vi "Teleop.vi"(10 "Match Info":T1={"Autonomous Elapsed Seconds"=0.0, "TeleOp Elapsed Seconds"=0.0, "Disabled Elapsed Seconds"=0.0, "Visited Autonomous"=FALSE, "Visited TeleOp"=FALSE, "Visited Disabled"=FALSE, "Autonomous Settings"={"Autonomous Style"=enum."Independent", "VI Refnum"=refnum}}, 11 "Call Context":T2) -> ()   [LabVIEW 2013]
doc: "This VI is called for each TeleOp packet received from the DS where the robot is not disabled. It is often used to read from the joysticks and update I/O or to update setpoints for timed control loops. It should complete and return within 20 milliseconds or it may miss DS packets."
uses:
  <vilib>/Rock Robotics/WPI/DriverStation/WPI_DriverStationDerivedRobotMode.ctl
  <vilib>/Rock Robotics/WPI/DriverStation/WPI_DriverStationMatch Info.ctl
  Robot Global Data.vi
  <vilib>/Rock Robotics/WPI/Joystick/WPI_JoystickGetSetRefNum.vi
  <vilib>/Rock Robotics/WPI/RobotDrive/WPI_RobotDriveMecanumDrive_Cartesian.vi
panel:
  in  "slow mode turn multiplier":dbl(knob)=0.5 scale=0.0..1.0
  in  "Deadzone":dbl=0.05
  out "Numeric 1":dbl(slide) scale=0.0..100.0
  out "Boolean 2":bool
  out "Boolean 1":bool
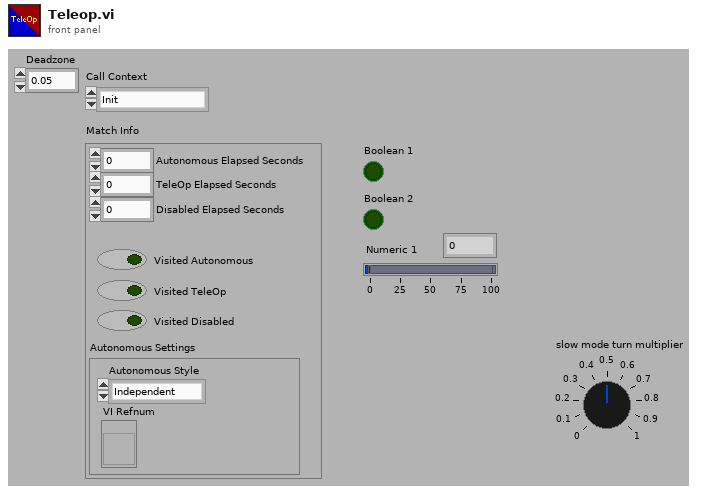
[diagram p1: front panel]
types:
  T1 = typedef "WPI_DriverStationMatch Info.ctl" = cluster{"Autonomous Elapsed Seconds":dbl, "TeleOp Elapsed Seconds":dbl, "Disabled Elapsed Seconds":dbl, "Visited Autonomous":bool, "Visited TeleOp":bool, "Visited Disabled":bool, "Autonomous Settings":cluster{"Autonomous Style":enum16{"Iterative", "Independent"}, "VI Refnum":refnum<vi>}}
  T2 = typedef "WPI_DriverStationDerivedRobotMode.ctl" = enum16{"Init", "Execute", "Stop"}
  T3 = typedef "WPI_JoystickDevRef.ctl" = cluster{"Device":T4}
  T4 = typedef "WPI_JoystickDeviceEnum.ctl" = enum16{"USB 1", "USB 2", "USB 3", "USB 4", "Kinect 1", "Kinect 2"}
  T5 = typedef "WPI_JoystickButtonState.ctl" = cluster{"Button 1":bool, "Button 2":bool, "Button 3":bool, "Button 4":bool, "Button 5":bool, "Button 6":bool, "Button 7":bool, "Button 8":bool, "Button 9":bool, "Button 10":bool, "Button 11":bool, "Button 12":bool}
  T6 = cluster{"axis 1 (x)":dbl, "axis 2 (y)":dbl, "axis 3 (throttle)":dbl, "axis 4":dbl, "axis 5":dbl, "axis 6":dbl}
  T7 = typedef "WPI_RobotDriveDevRef.ctl" = cluster{"DevStatus":errorcluster, "Motors[]":T8[], "Square Inputs":bool, "Max Output":dbl, "Isochronous":bool}
  T8 = typedef "WPI_MotorControlDeviceRef.ctl" = cluster{"DeviceStatus":errorcluster, "Type":enum16{"PWM", "CAN"}, "PWM":cluster{"Digital Module":T9, "PWM Channel":T10, "DeadBand":T11}, "CAN":cluster{"Device Number":u8, "Control Mode":T12, "Semaphore":T13, "Max Vout":dbl}, "Invert":bool, "TransformRef":T14, "InvTransformRef":T14}
  T9 = typedef "FPGA_TypedefDigitalModule.ctl" = enum16{"Digital Module 1", "Digital Module 2"}
  T10 = typedef "FPGA_DIOPWMChannel.ctl" = enum8{"PWM 1", "PWM 2", "PWM 3", "PWM 4", "PWM 5", "PWM 6", "PWM 7", "PWM 8", "PWM 9", "PWM 10", "Invalid"}
  T11 = typedef "WPI_PWMDeadband.ctl" = cluster{"Name":string, "maxPositivePwm":i32, "minPositivePwm":i32, "centerPwm":i32, "maxNegativePwm":i32, "minNegativePwm":i32, "angularRange":u16}
  T12 = typedef "WPI_CANJaguar_ControlMode.ctl" = enum8{"Percent VBus", "Current", "Speed", "Position", "Voltage"}
  T13 = typedef "Semaphore RefNum" = refnum<k1>
  T14 = typedef "WPI_PWMTransform_ConPane.ctl" = refnum<vi>
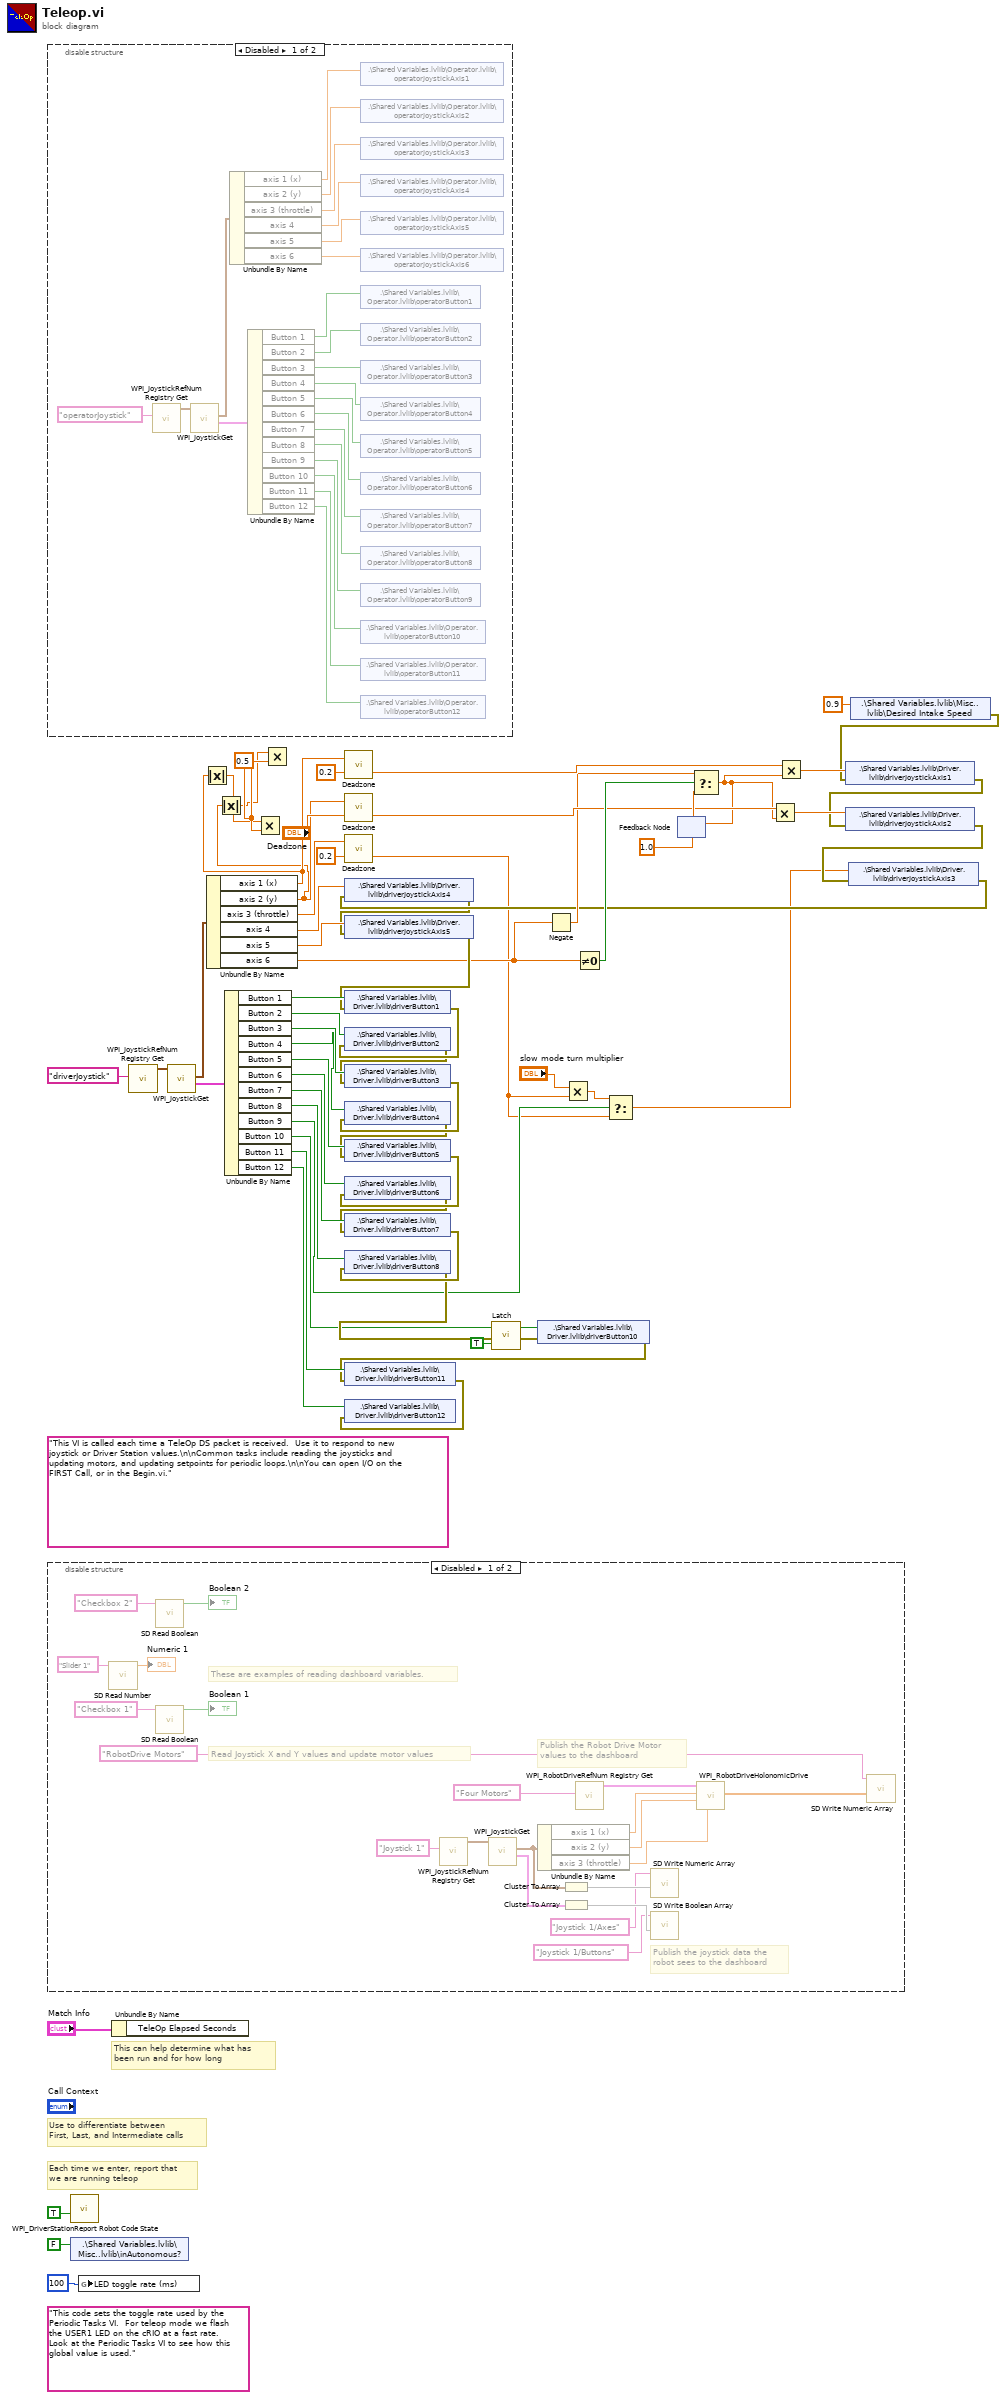
[diagram p0: block diagram]
diagram:
  w4 = 0.5 ("y")
  (unwired) "This code sets the toggle rate used by the Periodic Tasks VI.  For teleop mode we flash the USER1 LED on the cRIO at a fast rate.  Look at the Periodic Tasks VI to see how this global value is used."
  (unwired) "This VI is called each time a TeleOp DS packet is received.  Use it to respond to new joystick or Driver Station values.\n\nCommon tasks include reading the joysticks and updating motors, and updating setpoints for periodic loops.\n\nYou can open I/O on the FIRST Call, or in the Begin.vi."
  # "Each time we enter, report that\nwe are running teleop"
  # "Use to differentiate between\nFirst, Last, and Intermediate calls"
  # "This can help determine what has\nbeen run and for how long"
  n1 = disable-structure shown="Disabled" {
    frame Disabled {
      n2 = call <vilib>:"WPI_JoystickRefNum Registry Get.vi"("refnum name"="operatorJoystick") -> ("JoystickDevRef"=w85:T3)  [unwired: 9 in, 1 out]
      n3 = call <vilib>:"WPI_JoystickGet.vi"("JoystickDevRef"=w85) -> ("Buttons"=w83:T5, "Axes"=w84:T6)  [unwired: 4 in, 1 out]
      n4 = Unbundle By Name(w84) -> ("axis 1 (x)"=w82:dbl, "axis 2 (y)"=w81:dbl, "axis 3 (throttle)"=w80:dbl, "axis 4"=w79:dbl, "axis 5"=w78:dbl, "axis 6"=w77:dbl)
      n5 = Unbundle By Name(w83) -> ("Button 1"=w76:bool, "Button 2"=w75:bool, "Button 3"=w74:bool, "Button 4"=w73:bool, "Button 5"=w72:bool, "Button 6"=w71:bool, "Button 7"=w70:bool, "Button 8"=w69:bool, "Button 9"=w68:bool, "Button 10"=w67:bool, "Button 11"=w66:bool, "Button 12"=w65:bool)
      n6 = shared-variable ".\\Shared Variables.lvlib\\Operator.lvlib\\operatorJoystickAxis1"(w82) -> ()  [unwired: 1 in, 1 out]
      n7 = shared-variable ".\\Shared Variables.lvlib\\Operator.lvlib\\operatorJoystickAxis2"(w81) -> ()  [unwired: 1 in, 1 out]
      n8 = shared-variable ".\\Shared Variables.lvlib\\Operator.lvlib\\operatorJoystickAxis3"(w80) -> ()  [unwired: 1 in, 1 out]
      n9 = shared-variable ".\\Shared Variables.lvlib\\Operator.lvlib\\operatorJoystickAxis4"(w79) -> ()  [unwired: 1 in, 1 out]
      n10 = shared-variable ".\\Shared Variables.lvlib\\Operator.lvlib\\operatorJoystickAxis5"(w78) -> ()  [unwired: 1 in, 1 out]
      n11 = shared-variable ".\\Shared Variables.lvlib\\Operator.lvlib\\operatorJoystickAxis6"(w77) -> ()  [unwired: 1 in, 1 out]
      n12 = shared-variable ".\\Shared Variables.lvlib\\Operator.lvlib\\operatorButton1"(w76) -> ()  [unwired: 1 in, 1 out]
      n13 = shared-variable ".\\Shared Variables.lvlib\\Operator.lvlib\\operatorButton2"(w75) -> ()  [unwired: 1 in, 1 out]
      n14 = shared-variable ".\\Shared Variables.lvlib\\Operator.lvlib\\operatorButton3"(w74) -> ()  [unwired: 1 in, 1 out]
      n15 = shared-variable ".\\Shared Variables.lvlib\\Operator.lvlib\\operatorButton4"(w73) -> ()  [unwired: 1 in, 1 out]
      n16 = shared-variable ".\\Shared Variables.lvlib\\Operator.lvlib\\operatorButton5"(w72) -> ()  [unwired: 1 in, 1 out]
      n17 = shared-variable ".\\Shared Variables.lvlib\\Operator.lvlib\\operatorButton6"(w71) -> ()  [unwired: 1 in, 1 out]
      n18 = shared-variable ".\\Shared Variables.lvlib\\Operator.lvlib\\operatorButton7"(w70) -> ()  [unwired: 1 in, 1 out]
      n19 = shared-variable ".\\Shared Variables.lvlib\\Operator.lvlib\\operatorButton8"(w69) -> ()  [unwired: 1 in, 1 out]
      n20 = shared-variable ".\\Shared Variables.lvlib\\Operator.lvlib\\operatorButton9"(w68) -> ()  [unwired: 1 in, 1 out]
      n21 = shared-variable ".\\Shared Variables.lvlib\\Operator.lvlib\\operatorButton10"(w67) -> ()  [unwired: 1 in, 1 out]
      n22 = shared-variable ".\\Shared Variables.lvlib\\Operator.lvlib\\operatorButton11"(w66) -> ()  [unwired: 1 in, 1 out]
      n23 = shared-variable ".\\Shared Variables.lvlib\\Operator.lvlib\\operatorButton12"(w65) -> ()  [unwired: 1 in, 1 out]
    }
    frame Enabled {
    }
  }
  n24 = disable-structure shown="Disabled" {
    frame Disabled {
      # "These are examples of reading dashboard variables."
      # "Publish the Robot Drive Motor\nvalues to the dashboard"
      # "Publish the joystick data the\nrobot sees to the dashboard"
      # "Read Joystick X and Y values and update motor values"
      n25 = call <vilib>:"SD Read Number.vi"("Name"="Slider 1" ("refnum name")) -> ("Numeric"=→"Numeric 1":dbl)  [unwired: 8 in, 2 out]
      n26 = call <vilib>:"SD Read Boolean.vi"("Name"="Checkbox 2" ("refnum name")) -> ("Boolean"=→"Boolean 2":bool)  [unwired: 8 in, 2 out]
      n27 = call <vilib>:"SD Read Boolean.vi"("Name"="Checkbox 1" ("refnum name")) -> ("Boolean"=→"Boolean 1":bool)  [unwired: 8 in, 2 out]
      n28 = call <vilib>:"WPI_JoystickRefNum Registry Get.vi"("refnum name"="Joystick 1") -> ("JoystickDevRef"=w102:T3)  [unwired: 1 in, 9 out]
      n29 = call <vilib>:"WPI_JoystickGet.vi"("JoystickDevRef"=w102) -> ("Buttons"=w101:T5, "Axes"=w98:T6)  [unwired: 1 in, 4 out]
      n30 = Unbundle By Name(w98) -> ("axis 1 (x)"=w105:dbl, "axis 2 (y)"=w104:dbl, "axis 3 (throttle)"=w87:dbl)
      n31 = Cluster To Array(cluster=w98) -> (array=w97:dbl[])
      n32 = Cluster To Array(cluster=w101) -> (array=w100:bool[])
      n33 = call <vilib>:"WPI_RobotDriveRefNum Registry Get.vi"("refnum name"="Four Motors") -> ("RobotDriveDevRef"=w106:T7)  [unwired: 1 in, 9 out]
      n34 = call <vilib>:"SD Write Numeric Array.vi"("Numeric Array"=w97, "Name"="Joystick 1/Axes") -> ()  [unwired: 8 in, 2 out]
      n35 = call <vilib>:"SD Write Boolean Array.vi"("Boolean Array"=w100, "Name"="Joystick 1/Buttons") -> ()  [unwired: 8 in, 2 out]
      n36 = call-poly <vilib>:"WPI_RobotDriveHolonomicDrive.vi"("Rotation"=w87, "Y"=w104, "X"=w105, "RobotDriveDevRef"=w106) -> ("Motor Values"=w94:dbl[])  [unwired: 5 in, 2 out]
      n37 = call <vilib>:"SD Write Numeric Array.vi"("Numeric Array"=w94, "Name"="RobotDrive Motors") -> ()  [unwired: 8 in, 2 out]
    }
    frame Enabled {
    }
  }
  n38 = call <vilib>:"WPI_DriverStationReport Robot Code State.vi"("TeleOp"=TRUE ("Autonomous")) -> ()  [unwired: 10 in, 1 out]
  n39 = shared-variable ".\\Shared Variables.lvlib\\Misc..lvlib\\inAutonomous?"(FALSE ("inAutonomous?")) -> ()  [unwired: 1 in, 1 out]
  n40 = global write "Robot Global Data.vi" "LED toggle rate (ms)"(u32 100 ("LED ms toggle rate")) -> ()
  n41 = Unbundle By Name("Match Info") -> ()  [unwired: 1 out]
  n42 = call <vilib>:"WPI_JoystickRefNum Registry Get.vi"("refnum name"="driverJoystick") -> ("JoystickDevRef"=w60:T3)  [unwired: 9 in, 1 out]
  n43 = call <vilib>:"WPI_JoystickGet.vi"("JoystickDevRef"=w60) -> ("Buttons"=w58:T5, "Axes"=w59:T6)  [unwired: 4 in, 1 out]
  n44 = Unbundle By Name(w59) -> ("axis 1 (x)"=w6:dbl, "axis 2 (y)"=w5:dbl, "axis 3 (throttle)"=w44:dbl, "axis 4"=w48:dbl, "axis 5"=w47:dbl, "axis 6"=w25:dbl)
  n45 = Absolute Value(x=w6) -> (abs(x)=w3:dbl)
  n46 = Absolute Value(x=w5) -> (abs(x)=w2:dbl)
  n47 = Unbundle By Name(w58) -> ("Button 1"=w57:bool, "Button 2"=w56:bool, "Button 3"=w55:bool, "Button 4"=w8:bool, "Button 5"=w54:bool, "Button 6"=w53:bool, "Button 7"=w52:bool, "Button 8"=w51:bool, "Button 9"=w17:bool, "Button 10"=w12:bool, "Button 11"=w50:bool, "Button 12"=w49:bool)
  n48 = Multiply(x=w3, y=w4) -> ()  [unwired: 1 out]
  n49 = Multiply(x=w2, y=w4) -> ()  [unwired: 1 out]
  n50 = call "Deadzone.vi"("Deadzone"=0.2, "Input Signal"=w6) -> ("Output Signal"=w37:dbl)  [unwired: 1 out]
  n51 = call "Deadzone.vi"("Deadzone"="Deadzone", "Input Signal"=w5) -> ("Output Signal"=w40:dbl)  [unwired: 1 out]
  n52 = call "Deadzone.vi"("Deadzone"=0.2, "Input Signal"=w44) -> ("Output Signal"=w15:dbl)  [unwired: 1 out]
  n53 = call "Latch.vi"("Edge"=TRUE, "In"=w12) -> ("Out"=w11:bool)
  n54 = Negate(x=w25) -> (-x=w24:dbl)
  n55 = Multiply(x="slow mode turn multiplier", y=w15) -> (x*y=w16:dbl)
  n56 = Not Equal To 0?(x=w25) -> (x != 0?=w43:bool)
  n57 = Select(t=w16, s=w17, f=w15) -> (s? t:f=w13:dbl)
  n58 = feedback #1(1.0) -> (w42:dbl)
  n59 = Select(t=w24, s=w43, f=w42) -> (s? t:f=w38:dbl)
  n60 = feedback-in #1(w38) -> ()
  n61 = Multiply(x=w40, y=w38) -> (x*y=w39:dbl)
  n62 = Multiply(x=w37, y=w38) -> (x*y=w36:dbl)
  n63 = shared-variable ".\\Shared Variables.lvlib\\Misc..lvlib\\Desired Intake Speed"(0.9 ("Desired Intake Speed")) -> (error out=w9:errorcluster)  [unwired: 1 in]
  n64 = shared-variable ".\\Shared Variables.lvlib\\Driver.lvlib\\driverJoystickAxis1"(w36, error in=w9) -> (error out=w21:errorcluster)
  n65 = shared-variable ".\\Shared Variables.lvlib\\Driver.lvlib\\driverJoystickAxis2"(w39, error in=w21) -> (error out=w20:errorcluster)
  n66 = shared-variable ".\\Shared Variables.lvlib\\Driver.lvlib\\driverJoystickAxis3"(w13, error in=w20) -> (error out=w19:errorcluster)
  n67 = shared-variable ".\\Shared Variables.lvlib\\Driver.lvlib\\driverJoystickAxis4"(w48, error in=w19) -> (error out=w18:errorcluster)
  n68 = shared-variable ".\\Shared Variables.lvlib\\Driver.lvlib\\driverJoystickAxis5"(w47, error in=w18) -> (error out=w35:errorcluster)
  n69 = shared-variable ".\\Shared Variables.lvlib\\Driver.lvlib\\driverButton1"(w57, error in=w35) -> (error out=w34:errorcluster)
  n70 = shared-variable ".\\Shared Variables.lvlib\\Driver.lvlib\\driverButton2"(w56, error in=w34) -> (error out=w33:errorcluster)
  n71 = shared-variable ".\\Shared Variables.lvlib\\Driver.lvlib\\driverButton3"(w55, error in=w33) -> (error out=w32:errorcluster)
  n72 = shared-variable ".\\Shared Variables.lvlib\\Driver.lvlib\\driverButton4"(w8, error in=w32) -> (error out=w31:errorcluster)
  n73 = shared-variable ".\\Shared Variables.lvlib\\Driver.lvlib\\driverButton5"(w54, error in=w31) -> (error out=w30:errorcluster)
  n74 = shared-variable ".\\Shared Variables.lvlib\\Driver.lvlib\\driverButton6"(w53, error in=w30) -> (error out=w29:errorcluster)
  n75 = shared-variable ".\\Shared Variables.lvlib\\Driver.lvlib\\driverButton7"(w52, error in=w29) -> (error out=w28:errorcluster)
  n76 = shared-variable ".\\Shared Variables.lvlib\\Driver.lvlib\\driverButton8"(w51, error in=w28) -> (error out=w22:errorcluster)
  n77 = shared-variable ".\\Shared Variables.lvlib\\Driver.lvlib\\driverButton10"(w11, error in=w22) -> (error out=w27:errorcluster)
  n78 = shared-variable ".\\Shared Variables.lvlib\\Driver.lvlib\\driverButton11"(w50, error in=w27) -> (error out=w26:errorcluster)
  n79 = shared-variable ".\\Shared Variables.lvlib\\Driver.lvlib\\driverButton12"(w49, error in=w26) -> ()  [unwired: 1 out]
